vi "raster_scan_ground_shutter.vi"() -> ()   [LabVIEW 2013] (continued)
{"X"=1457.6770649491443, "Y"=0.9792905053235327}, {"X"=1458.7651269479165, "Y"=0.9823983446252466}, {"X"=1459.852974542116, "Y"=0.9830967304675241}, {"X"=1460.940607795108, "Y"=0.9785842230164021}, {"X"=1462.028026770236, "Y"=0.9775206880062371}, {"X"=1463.115231530815, "Y"=0.9787503056220913}, {"X"=1464.202222140141, "Y"=0.9797214290953251}, {"X"=1465.2889986614769, "Y"=0.9803641753236642}, {"X"=1466.3755611580664, "Y"=0.9821036191583837}, {"X"=1467.4619096931274, "Y"=0.978539694688825}, {"X"=1468.5480443298516, "Y"=0.9773624617620339}, {"X"=1469.6339651314086, "Y"=0.9807006551949096}, {"X"=1470.7196721609382, "Y"=0.9776792021711804}, {"X"=1471.8051654815604, "Y"=0.9801405710958422}, {"X"=1472.890445156365, "Y"=0.9788422567581777}, {"X"=1473.9755112484265, "Y"=0.9756071162075614}, {"X"=1475.0603638207806, "Y"=0.978305664540015}, {"X"=1476.1450029364496, "Y"=0.9757156870540381}, {"X"=1477.22942865843, "Y"=0.9787686258373013}, {"X"=1478.3136410496857, "Y"=0.9792534443330937}, {"X"=1479.3976401731636, "Y"=0.9761811767701299}, {"X"=1480.481426091784, "Y"=0.9801149830678351}, {"X"=1481.5649988684393, "Y"=0.9756151228933025}, {"X"=1482.6483585660003, "Y"=0.9791892417960691}, {"X"=1483.7315052473118, "Y"=0.9784822075875651}, {"X"=1484.8144389751922, "Y"=0.9803761026749522}, {"X"=1485.897159812443, "Y"=0.9794142210541505}, {"X"=1486.979667821831, "Y"=0.9777454282868382}, {"X"=1488.061963066103, "Y"=0.9765603212009248}, {"X"=1489.1440456079827, "Y"=0.9793187588636386}, {"X"=1490.2259155101667, "Y"=0.9805922827534587}, {"X"=1491.3075728353247, "Y"=0.9764488211952385}, {"X"=1492.3890176461057, "Y"=0.9783557981039106}, {"X"=1493.4702500051358, "Y"=0.9797315485802368}, {"X"=1494.5512699750122, "Y"=0.9776150196125559}, {"X"=1495.6320776183086, "Y"=0.9776877216361516}, {"X"=1496.712672997573, "Y"=0.9781695891128918}, {"X"=1497.7930561753328, "Y"=0.9738031398956338}, {"X"=1498.8732272140865, "Y"=0.975976844601347}, {"X"=1499.9531861763096, "Y"=0.9765304998861686}, {"X"=1501.0329331244568, "Y"=0.976932896128674}, {"X"=1502.1124681209478, "Y"=0.9800966831480284}, {"X"=1503.1917912281933, "Y"=0.9768824769343718}, {"X"=1504.2709025085678, "Y"=0.981309584860133}, {"X"=1505.3498020244213, "Y"=0.9788112290408383}, {"X"=1506.428489838087, "Y"=0.9749607521239584}, {"X"=1507.5069660118672, "Y"=0.9776436670703931}, {"X"=1508.5852306080433, "Y"=0.9781728498905934}, {"X"=1509.6632836888655, "Y"=0.9785040924428975}, {"X"=1510.7411253165735, "Y"=0.9808588594145039}, {"X"=1511.818755553368, "Y"=0.9802873517212242}, {"X"=1512.8961744614323, "Y"=0.9775486080858491}, {"X"=1513.973382102924, "Y"=0.9767280155604918}, {"X"=1515.0503785399785, "Y"=0.980209272149509}, {"X"=1516.1271638347032, "Y"=0.9800164628111341}, {"X"=1517.2037380491815, "Y"=0.9779781472644876}, {"X"=1518.2801012454781, "Y"=0.9801492617966195}, {"X"=1519.356253485624, "Y"=0.9786930631958413}, {"X"=1520.4321948316335, "Y"=0.9758135531220278}, {"X"=1521.507925345497, "Y"=0.9754907725499357}, {"X"=1522.5834450891723, "Y"=0.9781765485055535}, {"X"=1523.658754124602, "Y"=0.9787103618067179}, {"X"=1524.7338525137006, "Y"=0.9795724169903677}, {"X"=1525.8087403183565, "Y"=0.980684893431184}, {"X"=1526.8834176004366, "Y"=0.9771208914998462}, {"X"=1527.9578844217835, "Y"=0.9775073160780532}, {"X"=1529.032140844212, "Y"=0.9797555776149712}, {"X"=1530.10618692952, "Y"=0.975841176234859}, {"X"=1531.1800227394758, "Y"=0.9807727653780394}, {"X"=1532.2536483358228, "Y"=0.9802961901132733}, {"X"=1533.3270637802827, "Y"=0.9777395500524853}, {"X"=1534.400269134551, "Y"=0.9778205116075891}, {"X"=1535.4732644603034, "Y"=0.9790625062938085}, {"X"=1536.5460498191853, "Y"=0.9768981763432918}, {"X"=1537.6186252728232, "Y"=0.9786665184806389}, {"X"=1538.6909908828147, "Y"=0.9778748148771911}, {"X"=1539.7631467107403, "Y"=0.9774185537903284}, {"X"=1540.835092818148, "Y"=0.9794422669553383}, {"X"=1541.9068292665686, "Y"=0.9768522710498364}, {"X"=1542.9783561175022, "Y"=0.9779311791789327}, {"X"=1544.049673432434, "Y"=0.9777348271764831}, {"X"=1545.1207812728164, "Y"=0.9788311883596232}, {"X"=1546.1916797000786, "Y"=0.9801137926376271}, {"X"=1547.2623687756357, "Y"=0.9788638301844342}, {"X"=1548.3328485608647, "Y"=0.9773351540658165}, {"X"=1549.4031191171293, "Y"=0.9784129460538136}, {"X"=1550.473180505765, "Y"=0.9773105555519682}, {"X"=1551.543032788081, "Y"=0.9756165586699904}, {"X"=1552.6126760253678, "Y"=0.9806566212357941}, {"X"=1553.6821102788865, "Y"=0.9776974839417673}, {"X"=1554.7513356098798, "Y"=0.9798533480947225}, {"X"=1555.8203520795637, "Y"=0.9773735991839198}, {"X"=1556.8891597491306, "Y"=0.9781065565190785}, {"X"=1557.957758679745, "Y"=0.9791812863307896}, {"X"=1559.0261489325553, "Y"=0.976934001594789}, {"X"=1560.0943305686806, "Y"=0.9798934119983503}, {"X"=1561.1623036492178, "Y"=0.9797080714150074}, {"X"=1562.2300682352377, "Y"=0.9804595704839962}, {"X"=1563.2976243877897, "Y"=0.9780169362249083}, {"X"=1564.3649721679012, "Y"=0.9799845623788633}, {"X"=1565.432111636574, "Y"=0.9776505523367032}, {"X"=1566.4990428547812, "Y"=0.9786612468271689}, {"X"=1567.5657658834812, "Y"=0.9809144110707856}, {"X"=1568.6322807835995, "Y"=0.9757405630183322}, {"X"=1569.6985876160466, "Y"=0.9785541452864821}, {"X"=1570.7646864416984, "Y"=0.9818847727133657}, {"X"=1571.8305773214217, "Y"=0.9779227856602232}, {"X"=1572.896260316045, "Y"=0.9793508481684556}, {"X"=1573.9617354863833, "Y"=0.980887808587657}, {"X"=1575.027002893221, "Y"=0.9797121999265395}, {"X"=1576.0920625973235, "Y"=0.9795556996545292}, {"X"=1577.15691465943, "Y"=0.9766550361895545}, {"X"=1578.2215591402578, "Y"=0.9759789556077555}, {"X"=1579.2859961004988, "Y"=0.9815908904755111}, {"X"=1580.35022560082, "Y"=0.9785937882250549}, {"X"=1581.41424770187, "Y"=0.9819645665279645}, {"X"=1582.4780624642708, "Y"=0.979843167597932}, {"X"=1583.5416699486182, "Y"=0.9792802489088565}, {"X"=1584.6050702154869, "Y"=0.9790060313862785}, {"X"=1585.6682633254293, "Y"=0.9784271844295911}, {"X"=1586.7312493389722, "Y"=0.9784361245927183}, {"X"=1587.7940283166165, "Y"=0.9775708937146439}, {"X"=1588.856600318845, "Y"=0.9789041946582772}, {"X"=1589.9189654061154, "Y"=0.9774768633003437}, {"X"=1590.9811236388587, "Y"=0.9798817299531287}, {"X"=1592.0430750774847, "Y"=0.9768271507913547}, {"X"=1593.1048197823789, "Y"=0.9787911807962866}, {"X"=1594.1663578139055, "Y"=0.9783715358577475}, {"X"=1595.2276892324023, "Y"=0.9788361535376178}, {"X"=1596.2888140981859, "Y"=0.9793765834786251}, {"X"=1597.3497324715445, "Y"=0.9779362720028634}, {"X"=1598.410444412753, "Y"=0.9795457056765116}, {"X"=1599.4709499820517, "Y"=0.9797067699371061}, {"X"=1600.531249239662, "Y"=0.9808534483691963}, {"X"=1601.591342245785, "Y"=0.9781878073830106}, {"X"=1602.651229060596, "Y"=0.9802554323683685}, {"X"=1603.7109097442426, "Y"=0.9776897881450424}, {"X"=1604.7703843568543, "Y"=0.9797514273601062}, {"X"=1605.829652958537, "Y"=0.9789968213957626}, {"X"=1606.888715609371, "Y"=0.9786680583172949}, {"X"=1607.9475723694147, "Y"=0.9781996662549933}, {"X"=1609.006223298702, "Y"=0.9799905582549356}, {"X"=1610.0646684572441, "Y"=0.9801584266392093}, {"X"=1611.1229079050315, "Y"=0.9808165915061069}, {"X"=1612.1809417020254, "Y"=0.980629963941835}, {"X"=1613.2387699081667, "Y"=0.9779217757054299}, {"X"=1614.2963925833749, "Y"=0.980291231246423}, {"X"=1615.353809787546, "Y"=0.9802126966035473}, {"X"=1616.4110215805492, "Y"=0.9806800387009521}, {"X"=1617.468028022235, "Y"=0.9825340406943407}, {"X"=1618.5248291724251, "Y"=0.9788256639790675}, {"X"=1619.5814250909243, "Y"=0.9802906842015114}, {"X"=1620.637815837509, "Y"=0.979685976141551}, {"X"=1621.6940014719337, "Y"=0.9800339027601165}, {"X"=1622.7499820539335, "Y"=0.9779521660841378}, {"X"=1623.8057576432159, "Y"=0.9793762038551321}, {"X"=1624.8613282994656, "Y"=0.9785756484834109}, {"X"=1625.9166940823447, "Y"=0.9772795374000064}, {"X"=1626.971855051495, "Y"=0.9780014724416649}, {"X"=1628.0268112665321, "Y"=0.9769491921287421}, {"X"=1629.0815627870463, "Y"=0.981333694440951}, {"X"=1630.136109672612, "Y"=0.9784390781431715}, {"X"=1631.1904519827697, "Y"=0.9790742732109099}, {"X"=1632.2445897770504, "Y"=0.9796612246815406}, {"X"=1633.2985231149485, "Y"=0.9779598916744058}, {"X"=1634.3522520559459, "Y"=0.9772464628134946}, {"X"=1635.4057766594958, "Y"=0.9793400653452339}, {"X"=1636.4590969850296, "Y"=0.9797116577597221}, {"X"=1637.5122130919533, "Y"=0.9797059940747953}, {"X"=1638.5651250396568, "Y"=0.9808562777149027}, {"X"=1639.6178328874985, "Y"=0.9790804555327355}, {"X"=1640.6703366948186, "Y"=0.9788362371686626}, {"X"=1641.722636520934, "Y"=0.9787844420078925}, {"X"=1642.7747324251397, "Y"=0.9794474398454981}, {"X"=1643.8266244667045, "Y"=0.9804131255057831}, {"X"=1644.878312704874, "Y"=0.9768249479329455}, {"X"=1645.9297971988753, "Y"=0.9799389865441378}, {"X"=1646.9810780079088, "Y"=0.9783432068536082}, {"X"=1648.0321551911518, "Y"=0.9775263305205893}, {"X"=1649.083028807763, "Y"=0.9787347803249032}, {"X"=1650.1336989168726, "Y"=0.9808567682226018}, {"X"=1651.184165577591, "Y"=0.9782522449877368}, {"X"=1652.2344288490056, "Y"=0.9789066233804873}, {"X"=1653.284488790181, "Y"=0.978399712160505}, {"X"=1654.334345460157, "Y"=0.9775518534383865}, {"X"=1655.3839989179503, "Y"=0.9776201692032794}, {"X"=1656.4334492225616, "Y"=0.9790505282699306}, {"X"=1657.4826964329582, "Y"=0.9791007362859836}, {"X"=1658.5317406080926, "Y"=0.9796289092089305}, {"X"=1659.5805818068911, "Y"=0.9802344480197129}, {"X"=1660.6292200882588, "Y"=0.9794118671835017}, {"X"=1661.6776555110757, "Y"=0.9769578407595142}, {"X"=1662.725888134202, "Y"=0.9796671523854356}, {"X"=1663.7739180164745, "Y"=0.9772899941448419}, {"X"=1664.8217452167003, "Y"=0.9789999657090263}, {"X"=1665.869369793676, "Y"=0.9793822552018605}, {"X"=1666.9167918061676, "Y"=0.9778192616893263}, {"X"=1667.9640113129212, "Y"=0.9777885231437959}, {"X"=1669.0110283726551, "Y"=0.9797417352632923}, {"X"=1670.0578430440723, "Y"=0.9809342630258361}, {"X"=1671.104455385848, "Y"=0.9779252084439294}, {"X"=1672.1508654566371, "Y"=0.9766078448496384}, {"X"=1673.1970733150715, "Y"=0.9799766985367611}, {"X"=1674.2430790197561, "Y"=0.9784335113759398}, {"X"=1675.2888826292817, "Y"=0.9792316725161806}, {"X"=1676.3344842022125, "Y"=0.976438469155643}, {"X"=1677.3798837970842, "Y"=0.9789431735090179}, {"X"=1678.4250814724203, "Y"=0.9784990647101345}, {"X"=1679.4700772867131, "Y"=0.9784634992400977}, {"X"=1680.5148712984362, "Y"=0.9757776031845267}, {"X"=1681.5594635660389, "Y"=0.9785753222902629}, {"X"=1682.603854147955, "Y"=0.9762430899631663}, {"X"=1683.648043102582, "Y"=0.9786154222348789}, {"X"=1684.6920304883088, "Y"=0.982601098721033}, {"X"=1685.735816363493, "Y"=0.9787598651333007}, {"X"=1686.779400786472, "Y"=0.9796236090165618}, {"X"=1687.8227838155622, "Y"=0.9807569854592928}, {"X"=1688.865965509057, "Y"=0.9777286147683862}, {"X"=1689.9089459252239, "Y"=0.979530268059855}, {"X"=1690.9517251223103, "Y"=0.9795518390335218}, {"X"=1691.9943031585465, "Y"=0.9762685981835564}, {"X"=1693.0366800921304, "Y"=0.9764990724345295}, {"X"=1694.0788559812445, "Y"=0.9793632033260535}, {"X"=1695.1208308840478, "Y"=0.9784431206603648}, {"X"=1696.162604858673, "Y"=0.9800970609348729}, {"X"=1697.204177963233, "Y"=0.9798274514050527}, {"X"=1698.2455502558198, "Y"=0.9767392079564985}, {"X"=1699.2867217945052, "Y"=0.9779580128194008}, {"X"=1700.3276926373287, "Y"=0.9756815094964185}, {"X"=1701.368462842319, "Y"=0.9800487876203458}, {"X"=1702.4090324674746, "Y"=0.9761434590853568}, {"X"=1703.4494015707742, "Y"=0.9778648023676554}, {"X"=1704.4895702101746, "Y"=0.9774400128118678}, {"X"=1705.5295384436095, "Y"=0.9787943730431603}, {"X"=1706.5693063289923, "Y"=0.978395003858087}, {"X"=1707.6088739242089, "Y"=0.9781690442984677}, {"X"=1708.6482412871314, "Y"=0.9768357067469553}, {"X"=1709.6874084756023, "Y"=0.9785722403014319}, {"X"=1710.7263755474444, "Y"=0.9794128983222802}, {"X"=1711.765142560456, "Y"=0.9762472144277007}, {"X"=1712.8037095724192, "Y"=0.980017853288302}, {"X"=1713.8420766410868, "Y"=0.9784777089298898}, {"X"=1714.8802438241908, "Y"=0.9788070467014609}, {"X"=1715.918211179447, "Y"=0.9777741715615405}, {"X"=1716.9559787645442, "Y"=0.9791586404821226}, {"X"=1717.9935466371467, "Y"=0.9797751943038832}, {"X"=1719.0309148548993, "Y"=0.9781731952451092}, {"X"=1720.068083475427, "Y"=0.9786903221799141}, {"X"=1721.1050525563276, "Y"=0.9772549072141031}, {"X"=1722.1418221551803, "Y"=0.9765150697236492}, {"X"=1723.1783923295413, "Y"=0.9773240982124607}, {"X"=1724.214763136945, "Y"=0.9791583881092693}, {"X"=1725.250934634904, "Y"=0.9784526724453544}, {"X"=1726.2869068809046, "Y"=0.9777962347228817}, {"X"=1727.3226799324184, "Y"=0.9780085659065672}, {"X"=1728.3582538468886, "Y"=0.9779903185671098}, {"X"=1729.393628681741, "Y"=0.9766604181863742}, {"X"=1730.428804494373, "Y"=0.9791432873661055}, {"X"=1731.4637813421655, "Y"=0.9798748523350176}, {"X"=1732.4985592824764, "Y"=0.9784743079655346}, {"X"=1733.5331383726434, "Y"=0.9784825300354543}, {"X"=1734.5675186699748, "Y"=0.9785467117994335}, {"X"=1735.6017002317642, "Y"=0.979534546347603}, {"X"=1736.6356831152796, "Y"=0.982177067294777}, {"X"=1737.6694673777704, "Y"=0.9797240911901233}, {"X"=1738.7030530764594, "Y"=0.9790253743667566}, {"X"=1739.7364402685507, "Y"=0.9815129154446102}, {"X"=1740.7696290112233, "Y"=0.980432858830974}, {"X"=1741.8026193616408, "Y"=0.9798457306402057}, {"X"=1742.835411376938, "Y"=0.9781409027568759}, {"X"=1743.868005114229, "Y"=0.9788862198138762}, {"X"=1744.9004006306095, "Y"=0.9757087423855413}, {"X"=1745.9325979831483, "Y"=0.9798092930085314}, {"X"=1746.9645972288977, "Y"=0.9789802741859566}, {"X"=1747.9963984248845, "Y"=0.9805471172994134}, {"X"=1749.0280016281145, "Y"=0.9785389300564209}, {"X"=1750.0594068955684, "Y"=0.9770374391897149}, {"X"=1751.0906142842127, "Y"=0.9775021384461788}, {"X"=1752.1216238509876, "Y"=0.9794676904895196}, {"X"=1753.152435652809, "Y"=0.9801654916078579}, {"X"=1754.183049746574, "Y"=0.9789424499526841}, {"X"=1755.2134661891573, "Y"=0.9770892255789045}, {"X"=1756.243685037413, "Y"=0.9776593168216676}, {"X"=1757.2737063481677, "Y"=0.9779906119034862}, {"X"=1758.3035301782381, "Y"=0.9781764711339365}, {"X"=1759.3331565844067, "Y"=0.9796097506756954}, {"X"=1760.3625856234391, "Y"=0.9788229781819409}, {"X"=1761.3918173520813, "Y"=0.9797000451931207}, {"X"=1762.4208518270536, "Y"=0.9772262704494723}, {"X"=1763.449689105058, "Y"=0.9793011383686007}, {"X"=1764.4783292427744, "Y"=0.9797462455262113}, {"X"=1765.5067722968568, "Y"=0.9790906455724389}, {"X"=1766.5350183239393, "Y"=0.9787694192292369}, {"X"=1767.5630673806413, "Y"=0.9773923919944699}, {"X"=1768.5909195235492, "Y"=0.9780613554354805}, {"X"=1769.6185748092373, "Y"=0.9753480333886292}, {"X"=1770.6460332942527, "Y"=0.9776669800733908}, {"X"=1771.6732950351213, "Y"=0.9774852126882629}, {"X"=1772.7003600883502, "Y"=0.9792762661382732}, {"X"=1773.727228510419, "Y"=0.9778884418100252}, {"X"=1774.7539003577956, "Y"=0.9758349135196726}, {"X"=1775.780375686917, "Y"=0.9790951870913759}, {"X"=1776.8066545542008, "Y"=0.9784810089527837}, {"X"=1777.832737016047, "Y"=0.9797035920414627}, {"X"=1778.8586231288302, "Y"=0.9794844663168093}, {"X"=1779.8843129489044, "Y"=0.9781376071318827}, {"X"=1780.9098065326032, "Y"=0.9750094677165442}, {"X"=1781.9351039362352, "Y"=0.9780984964063493}, {"X"=1782.9602052160903, "Y"=0.9754901241953642}, {"X"=1783.9851104284364, "Y"=0.9788789968076032}, {"X"=1785.0098196295219, "Y"=0.9761625032883274}, {"X"=1786.0343328755714, "Y"=0.977184310500348}, {"X"=1787.0586502227857, "Y"=0.9763453938178065}, {"X"=1788.0827717273478, "Y"=0.9792373851417304}, {"X"=1789.1066974454172, "Y"=0.9754176689748405}, {"X"=1790.1304274331344, "Y"=0.9787418979212442}, {"X"=1791.1539617466153, "Y"=0.9779537906626933}, {"X"=1792.1773004419586, "Y"=0.9783783911467727}, {"X"=1793.200443575237, "Y"=0.9777594296522633}, {"X"=1794.2233912025015, "Y"=0.9773798356027293}, {"X"=1795.2461433797885, "Y"=0.9772880946873316}, {"X"=1796.268700163103, "Y"=0.976721049350884}, {"X"=1797.291061608438, "Y"=0.9782575538452549}, {"X"=1798.3132277717596, "Y"=0.981480761676852}, {"X"=1799.3351987090107, "Y"=0.9767565408104497}, {"X"=1800.356974476123, "Y"=0.9764783426267764}, {"X"=1801.3785551289936, "Y"=0.9783902648770324}, {"X"=1802.3999407235092, "Y"=0.9785140953183166}, {"X"=1803.4211313155251, "Y"=0.9775113160777504}, {"X"=1804.4421269608847, "Y"=0.9785064598563911}, {"X"=1805.462927715407, "Y"=0.9778236195481496}, {"X"=1806.4835336348847, "Y"=0.9778192965434114}, {"X"=1807.503944775096, "Y"=0.978177936326559}, {"X"=1808.5241611917927, "Y"=0.9786243269548447}, {"X"=1809.5441829407114, "Y"=0.9795102802219587}, {"X"=1810.5640100775604, "Y"=0.977832296174399}, {"X"=1811.5836426580333, "Y"=0.9801041553279659}, {"X"=1812.6030807377952, "Y"=0.9787686082046061}, {"X"=1813.622324372498, "Y"=0.9762591413703259}, {"X"=1814.6413736177635, "Y"=0.9785764588841125}, {"X"=1815.6602285292006, "Y"=0.9778338211092795}, {"X"=1816.678889162394, "Y"=0.9786470411846112}, {"X"=1817.6973555729046, "Y"=0.9780455869984812}, {"X"=1818.7156278162763, "Y"=0.9772685688395546}, {"X"=1819.7337059480287, "Y"=0.9790073728881996}, {"X"=1820.7515900236604, "Y"=0.9776787156291022}, {"X"=1821.7692800986495, "Y"=0.981571042496983}, {"X"=1822.7867762284554, "Y"=0.9781551040759343}, {"X"=1823.8040784685134, "Y"=0.9775827328985149}, {"X"=1824.821186874237, "Y"=0.9790314094428728}, {"X"=1825.8381015010223, "Y"=0.97651494318833}, {"X"=1826.8548224042418, "Y"=0.98117111940764}, {"X"=1827.8713496392438, "Y"=0.9790448337557365}, {"X"=1828.8876832613619, "Y"=0.9792762568727814}, {"X"=1829.9038233259057, "Y"=0.9814170280977215}, {"X"=1830.9197698881605, "Y"=0.9769394138414527}, {"X"=1831.9355230033968, "Y"=0.9779927873623165}, {"X"=1832.9510827268593, "Y"=0.9795814602795806}, {"X"=1833.966449113775, "Y"=0.9813169438214728}, {"X"=1834.9816222193472, "Y"=0.9791962839304864}, {"X"=1835.9966020987592, "Y"=0.978443602610066}, {"X"=1837.0113888071735, "Y"=0.979330901923164}, {"X"=1838.025982399728, "Y"=0.9793733883949935}, {"X"=1839.040382931546, "Y"=0.9785176881927857}, {"X"=1840.0545904577286, "Y"=0.9787976042022226}, {"X"=1841.068605033351, "Y"=0.9794191523481688}, {"X"=1842.0824267134715, "Y"=0.9790665855910927}, {"X"=1843.0960555531262, "Y"=0.9783607833794199}, {"X"=1844.1094916073316, "Y"=0.981239000018723}, {"X"=1845.1227349310811, "Y"=0.9760725103032508}, {"X"=1846.1357855793499, "Y"=0.9802543813509697}, {"X"=1847.1486436070877, "Y"=0.9802118944100315}, {"X"=1848.1613090692265, "Y"=0.9788447902308257}, {"X"=1849.1737820206813, "Y"=0.9788741535108112}, {"X"=1850.1860625163386, "Y"=0.9797346774488815}, {"X"=1851.19815061107, "Y"=0.9769856196301054}, {"X"=1852.2100463597233, "Y"=0.979878008180614}, {"X"=1853.221749817122, "Y"=0.9761372153962043}, {"X"=1854.233261038079, "Y"=0.9790780443105339}, {"X"=1855.2445800773748, "Y"=0.9786918992409724}, {"X"=1856.2557069897791, "Y"=0.9783276499689203}, {"X"=1857.2666418300307, "Y"=0.9797503315777013}, {"X"=1858.2773846528562, "Y"=0.9776083716249421}, {"X"=1859.2879355129598, "Y"=0.9770551335500846}, {"X"=1860.2982944650225, "Y"=0.979004766786602}, {"X"=1861.3084615637028, "Y"=0.9799782313870046}, {"X"=1862.3184368636428, "Y"=0.9770803550491507}, {"X"=1863.3282204194622, "Y"=0.978975563881147}, {"X"=1864.337812285757, "Y"=0.9799645707401039}, {"X"=1865.3472125171106, "Y"=0.9801723270677862}, {"X"=1866.3564211680773, "Y"=0.9788358662998463}, {"X"=1867.3654382931952, "Y"=0.9765847371482588}, {"X"=1868.3742639469779, "Y"=0.9790676397118934}, {"X"=1869.3828981839238, "Y"=0.9812889246294414}, {"X"=1870.391341058503, "Y"=0.9774577161709844}, {"X"=1871.3995926251753, "Y"=0.980594262876655}, {"X"=1872.4076529383697, "Y"=0.9792702411654549}, {"X"=1873.4155220524979, "Y"=0.9790746036664525}, {"X"=1874.4232000219565, "Y"=0.9810852257689248}, {"X"=1875.4306869011118, "Y"=0.9795606590451479}, {"X"=1876.4379827443195, "Y"=0.9801611141715787}, {"X"=1877.4450876059084, "Y"=0.9786582015465105}, {"X"=1878.4520015401865, "Y"=0.9788312536969757}, {"X"=1879.4587246014419, "Y"=0.9795506376816854}, {"X"=1880.4652568439433, "Y"=0.9808280442755959}, {"X"=1881.4715983219419, "Y"=0.9782914192105046}, {"X"=1882.4777490896631, "Y"=0.9795263525003457}, {"X"=1883.4837092013126, "Y"=0.9802605203766053}, {"X"=1884.4894787110768, "Y"=0.9801816775097535}, {"X"=1885.4950576731223, "Y"=0.9801096012430007}, {"X"=1886.5004461415922, "Y"=0.9796802539288852}, {"X"=1887.5056441706138, "Y"=0.9788520860491313}, {"X"=1888.510651814289, "Y"=0.978659668379837}, {"X"=1889.5154691267023, "Y"=0.977015575532349}, {"X"=1890.5200961619184, "Y"=0.9787515604122116}, {"X"=1891.524532973976, "Y"=0.9768297562113655}, {"X"=1892.5287796169011, "Y"=0.9785475232918758}, {"X"=1893.5328361446932, "Y"=0.978116773405777}, {"X"=1894.5367026113352, "Y"=0.9811734737768301}, {"X"=1895.540379070785, "Y"=0.9804007166695333}, {"X"=1896.5438655769865, "Y"=0.9802706286345342}, {"X"=1897.547162183857, "Y"=0.9789474999633454}, {"X"=1898.5502689452985, "Y"=0.9764637671130718}, {"X"=1899.5531859151895, "Y"=0.9778795664386171}, {"X"=1900.5559131473867, "Y"=0.9784828326256647}, {"X"=1901.5584506957314, "Y"=0.9787769985370004}, {"X"=1902.5607986140392, "Y"=0.9798369721889083}, {"X"=1903.5629569561104, "Y"=0.9820482127941871}, {"X"=1904.5649257757213, "Y"=0.9785111601732347}, {"X"=1905.5667051266269, "Y"=0.9796830451602337}, {"X"=1906.5682950625664, "Y"=0.9787209677077426}, {"X"=1907.5696956372535, "Y"=0.98122288862003}, {"X"=1908.570906904389, "Y"=0.9809305064389832}, {"X"=1909.5719289176448, "Y"=0.9790387967034756}, {"X"=1910.5727617306782, "Y"=0.9794775159709218}, {"X"=1911.5734053971228, "Y"=0.9807386672057676}, {"X"=1912.573859970592, "Y"=0.9779631608593421}, {"X"=1913.574125504687, "Y"=0.9802046696643638}, {"X"=1914.5742020529756, "Y"=0.9780746838834492}, {"X"=1915.5740896690154, "Y"=0.9808649271816879}, {"X"=1916.573788406338, "Y"=0.9804333729213841}, {"X"=1917.5732983184594, "Y"=0.9801111109332562}, {"X"=1918.5726194588722, "Y"=0.9782040652735418}, {"X"=1919.5717518810488, "Y"=0.9791773277008486}, {"X"=1920.5706956384452, "Y"=0.9796555558287696}, {"X"=1921.5694507844885, "Y"=0.9789302800714461}, {"X"=1922.5680173725973, "Y"=0.9815528643924064}, {"X"=1923.566395456162, "Y"=0.9778044788192052}, {"X"=1924.5645850885558, "Y"=0.9783244097180387}, {"X"=1925.5625863231303, "Y"=0.9778964226146003}, {"X"=1926.5603992132171, "Y"=0.9787447398864959}, {"X"=1927.5580238121288, "Y"=0.9811759269001352}, {"X"=1928.5554601731558, "Y"=0.9798108032783646}, {"X"=1929.552708349572, "Y"=0.9798681796090567}, {"X"=1930.5497683946285, "Y"=0.9788799727761672}, {"X"=1931.5466403615578, "Y"=0.9788770140009356}, {"X"=1932.543324303568, "Y"=0.9799177632065718}, {"X"=1933.5398202738547, "Y"=0.9799634201036204}, {"X"=1934.5361283255868, "Y"=0.9798222448100651}, {"X"=1935.5322485119166, "Y"=0.9808393976744711}, {"X"=1936.528180885976, "Y"=0.9816005991663963}, {"X"=1937.523925500872, "Y"=0.97864600755322}, {"X"=1938.519482409702, "Y"=0.980309985973617}, {"X"=1939.5148516655336, "Y"=0.9781692490184501}, {"X"=1940.5100333214207, "Y"=0.9785093256720591}, {"X"=1941.5050274303896, "Y"=0.9799035052070364}, {"X"=1942.4998340454558, "Y"=0.9780111452063708}, {"X"=1943.4944532196087, "Y"=0.9817768573475947}, {"X"=1944.4888850058198, "Y"=0.9782104729191251}, {"X"=1945.483129457042, "Y"=0.979143828287662}, {"X"=1946.4771866262035, "Y"=0.9782644829264983}, {"X"=1947.471056566218, "Y"=0.97950360852036}, {"X"=1948.4647393299792, "Y"=0.9783169772597466}, {"X"=1949.4582349703528, "Y"=0.9798836359151304}, {"X"=1950.451543540196, "Y"=0.9791266953634022}, {"X"=1951.4446650923376, "Y"=0.9789837971330411}, {"X"=1952.4375996795911, "Y"=0.9813588982417887}, {"X"=1953.4303473547443, "Y"=0.9790520184393244}, {"X"=1954.422908170576, "Y"=0.9815722723554481}, {"X"=1955.415282179835, "Y"=0.9784927175757242}, {"X"=1956.4074694352523, "Y"=0.9788729195898936}, {"X"=1957.399469989544, "Y"=0.9791868614295317}, {"X"=1958.3912838953984, "Y"=0.9808439674180319}, {"X"=1959.382911205492, "Y"=0.9794424127876905}, {"X"=1960.3743519724785, "Y"=0.9811556122378184}, {"X"=1961.3656062489868, "Y"=0.9808021942940341}, {"X"=1962.3566740876313, "Y"=0.9800973819614038}, {"X"=1963.347555541011, "Y"=0.9795272574137769}, {"X"=1964.3382506616945, "Y"=0.9788140858856408}, {"X"=1965.3287595022373, "Y"=0.9780253232029532}, {"X"=1966.3190821151757, "Y"=0.979245748551627}, {"X"=1967.3092185530195, "Y"=0.9777558477121077}, {"X"=1968.2991688682703, "Y"=0.980276730191531}, {"X"=1969.288933113397, "Y"=0.9799821956293429}, {"X"=1970.2785113408574, "Y"=0.978955057838978}, {"X"=1971.2679036030884, "Y"=0.9823503552134017}, {"X"=1972.2571099525062, "Y"=0.9793230769314857}, {"X"=1973.246130441504, "Y"=0.9805669908359534}, {"X"=1974.234965122462, "Y"=0.9781158302205418}, {"X"=1975.223614047734, "Y"=0.9775909120825961}, {"X"=1976.212077269661, "Y"=0.979277706163912}, {"X"=1977.2003548405555, "Y"=0.9800070006509044}, {"X"=1978.1884468127198, "Y"=0.9795861716333901}, {"X"=1979.1763532384293, "Y"=0.977022092442501}, {"X"=1980.1640741699453, "Y"=0.9789258844658819}, {"X"=1981.1516096595064, "Y"=0.9792859180687412}, {"X"=1982.1389597593302, "Y"=0.9796248230956071}, {"X"=1983.1261245216187, "Y"=0.9804563919160044}, {"X"=1984.1131039985503, "Y"=0.979893234963858}, {"X"=1985.0998982422836, "Y"=0.9788294025328086}, {"X"=1986.086507304967, "Y"=0.9769723734116809}, {"X"=1987.0729312387155, "Y"=0.9783824752784152}, {"X"=1988.0591700956336, "Y"=0.9792177578466847}, {"X"=1989.0452239278025, "Y"=0.9788646746877344}, {"X"=1990.0310927872854, "Y"=0.9797103022782087}, {"X"=1991.0167767261282, "Y"=0.9786557517258911}, {"X"=1992.0022757963511, "Y"=0.9784247299328789}, {"X"=1992.987590049959, "Y"=0.9799351881103269}, {"X"=1993.9727195389369, "Y"=0.9801767642340488}, {"X"=1994.957664315253, "Y"=0.9791864057834342}, {"X"=1995.942424430849, "Y"=0.9806157724480351}, {"X"=1996.9269999376543, "Y"=0.9814342305423074}, {"X"=1997.9113908875738, "Y"=0.979347148988982}, {"X"=1998.8955973324953, "Y"=0.9787358726657928}, {"X"=1999.8796193242888, "Y"=0.9799108384264307}, {"X"=2000.8634569147994, "Y"=0.9801913761237805}, {"X"=2001.8471101558578, "Y"=0.9806815968287386}, {"X"=2002.8305790992738, "Y"=0.9791286421943739}]
  in  "# Images":u16=200 min=2 max=10000 step=2
  out "error out":errorcluster
  out "Camera Handle":u32=16842752
  out "Temperature":dbl=-75.5
  in  "error in":errorcluster
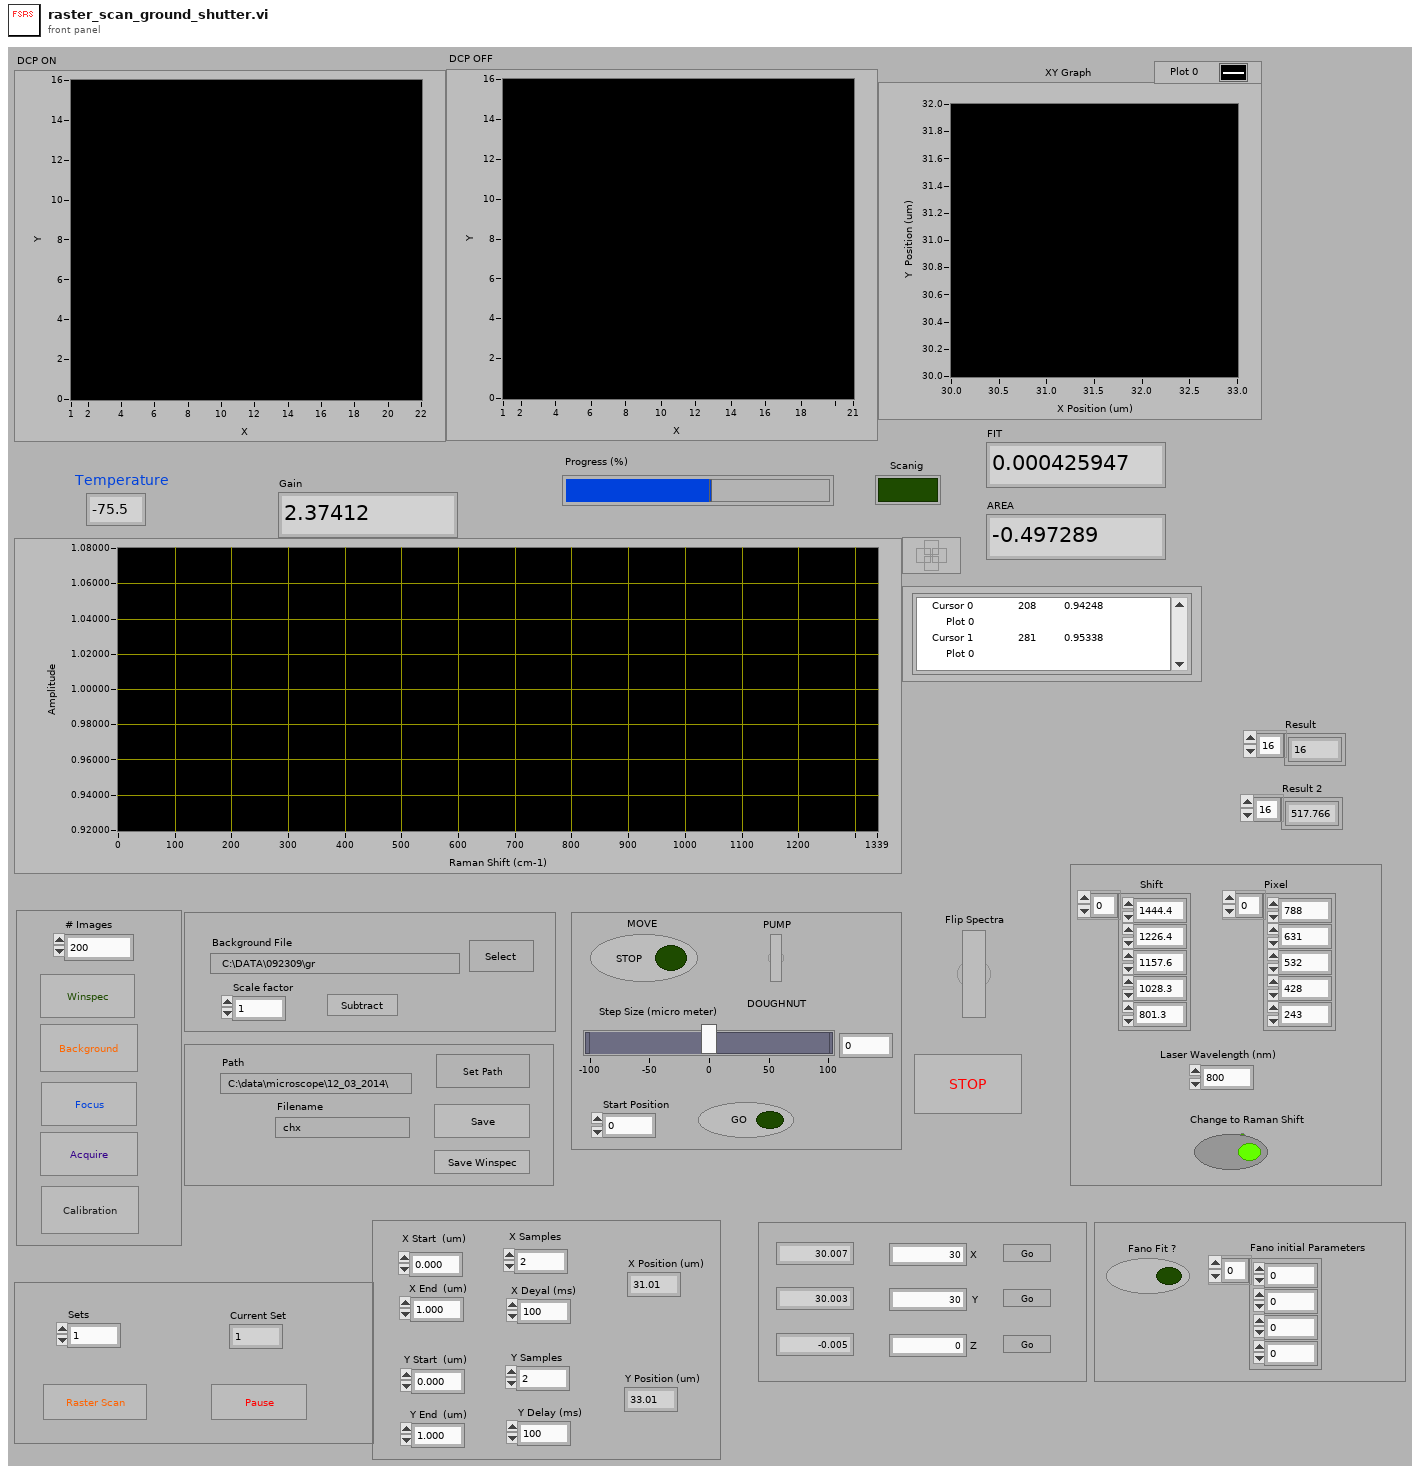
[diagram p1: front panel]
types:
  T1 = typedef "Control 2.ctl" = dbl[]
  T2 = cluster{"X start":u32, "X end":u32, "X Binning/Grouping":u32, "Y start":u32, "Y end":u32, "Y Binning/Grouping":u32}
  T3 = cluster{dbl[][], dbl[][], dbl[][], dbl[][], bool}
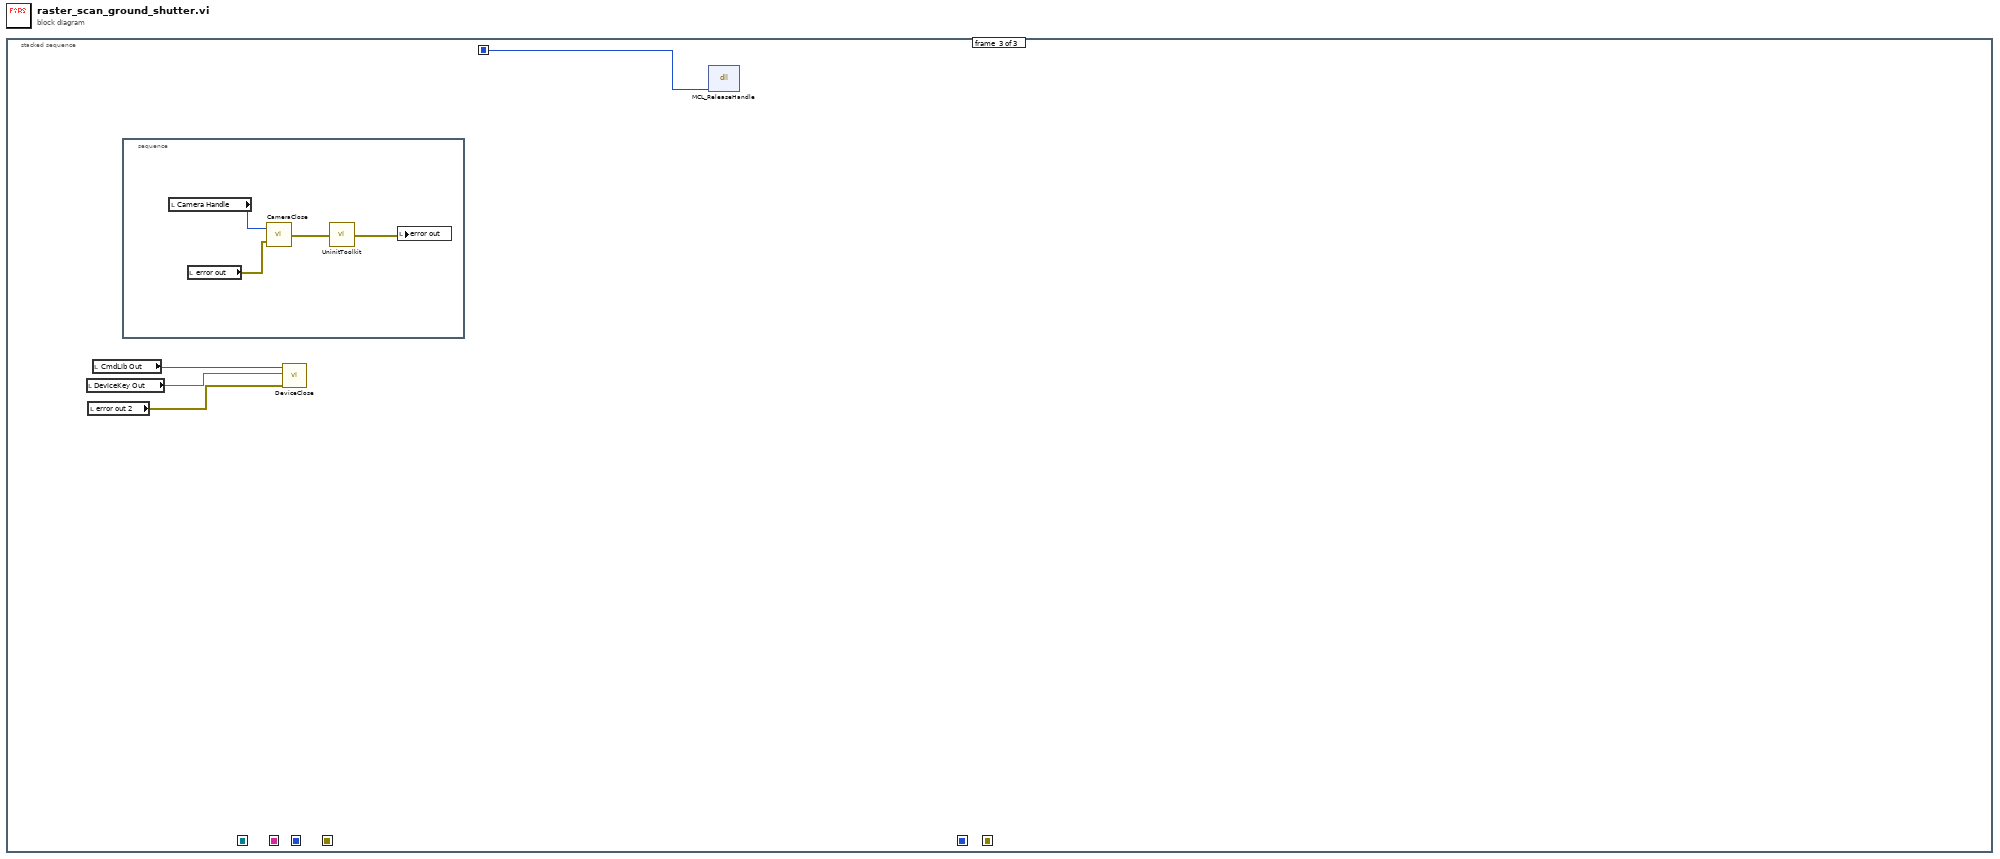
[diagram p0: block diagram]
diagram:
  n1 = stacked-sequence {
    seq-local: [w9 _ _] -> [_ w101 _]
    seq-local: [w8 _ _] -> [_ w100 _]
    seq-local: [w7 _ _] -> [_ w99 _]
    seq-local: [w6 _ _] -> [_ w98 _]
    seq-local: [w5 _ _] -> [_ w97 w744]
    seq-local: [w4 _ _] -> [_ w96 _]
    seq-local: [w3 _ _] -> [_ w95 _]
    frame #0 {
      w1 = 1340
      w67 = 0
      w69 = 8
      # "4: shutter opened while waiting for trigger\n3: Shutter opened during entire acq sequence\n2:Shutter opened and closed for each exposure\n\nOther numbers: Time in ms to open and close"
      # "1 is for free run, 3 ext sync"
      # "Parameter id settings:\n119: enable custon timing for horizontal and vertical shift\n121:Parallel shift time override\n146: Skip serial register clean\n 4:  Set logic output to \"Not Ready\" (necessary for chopper sync)"
      # "Setting up the PIXIS and all the environment variables\nHave Renee fill in the rest."
      n2 = call "ExSubInitNOpenCam.vi"("error in (no error)"="error in") -> ("Camera Handle"=w82:u32, "error out"=w39:errorcluster)
      n3 = call <userlib>:"CameraGetDataDim.vi"("Camera Handle"=w82, "error in"=w39) -> ("Camera Handle"=w79:u32, "Xdim"=w81:u32, "Ydim"=w80:u32, "error out"=w78:errorcluster)
      n4 = global write "MaxX.vi" "X Max in"(w81) -> ()
      n5 = global write "MaxY.vi" "Max Y in"(w80) -> ()
      n6 = call "pico_init.vi"() -> ("error out 3"=w6:errorcluster, "ID"=w7:i32, "key"=w8:string, "CmdLib Out"=w9:refnum<k24>)  [unwired: 8 in]
      n7 = call <userlib>:"CameraSetTemp.vi"("error in (no error)"=w78, "Temperature"=-75, "Camera Handle"=w79) -> ("error out"=w75:errorcluster, "Camera Handle"=w76:u32)
      n8 = call <userlib>:"CameraADCset.vi"("ADC offset"=0, "Read Out port"=2, "error in (no error)"=w75, "ADC Gain"=1, "ADC Speed"=-2, "Camera Handle"=w76) -> ("error out"=w70:errorcluster, "Camera Handle"=w71:u32)
      n9 = Bundle(w69, w69, 100, w67, w67, w1) -> (w66:cluster{i32, i32, i32, i32, i32, i32})  [unwired: 1 in]
      n10 = call <userlib>:"CameraSetCustomChip.vi"("error in (no error)"=w70, "Custom Chip Settings"=w66, "Enable/Disable Custom Chip"=TRUE, "Camera Handle"=w71) -> ("error out"=w63:errorcluster, "Camera Handle"=w64:u32)
      n11 = call <userlib>:"CameraSkips.vi"("Camera Handle"=w64, "Minimum Block Size"=100, "Number of Minimum blocks"=1, "error in"=w63, "Type of Skips"=1) -> ("Camera Handle"=w58:u32, "error out"=w59:errorcluster)
      n12 = call "StandardInit.vi"() -> ("Outgoing Handle"=w5:i32)  [unwired: 1 in]
      n13 = call <userlib>:"CameraCleans.vi"("Camera Handle"=w58, "Number of Clears"=1, "Number of Strips Per Clear"=100, "error in"=w59, "Continuous Clears"=0) -> ("Camera Handle"=w53:u32, "error out"=w54:errorcluster)
      n14 = call <userlib>:"CameraTrigger.vi"("error in"=w54, "Trigger Edge"=1, "Timing Mode"=3, "Camera Handle"=w53) -> ("error out"=w31:errorcluster, "Camera Handle"=w30:u32)
      n15 = Bundle By Name(cluster=T2 {"X start"=0, "X end"=0, "X Binning/Grouping"=0, "Y start"=0, "Y end"=0, "Y Binning/Grouping"=0} ("ROI Params"), "X start"=u32 1, "X end"=u32 1340, "X Binning/Grouping"=u32 1, "Y start"=u32 1, "Y end"=u32 100, "Y Binning/Grouping"=u32 100) -> (w12:T2)
      n16 = call <userlib>:"CameraROI.vi"("error in"=w31, "ROI Params"=w12, "ROI Index"=1, "Camera Handle"=w30) -> ("error out"=w25:errorcluster, "Camera Handle"=w24:u32)
      n17 = call <userlib>:"CameraShutter.vi"("Camera Handle"=w24, "Shutter Comp Time: Pre Open"=0, "Shutter Comp Time: Post Open"=0, "error in"=w25, "Shutter State"=3) -> ("Camera Handle"=w23:u32, "error out"=w14:errorcluster)
      n18 = call <userlib>:"CameraSetVar.vi"("error in"=w14, "Value"=1.0, "Parameter ID"=119, "Camera Handle"=w23) -> ("error out"=w48:errorcluster, "CameraHandle"=w46:u32)
      n19 = call <userlib>:"CameraSetVar.vi"("error in"=w48, "Value"=3200.0, "Parameter ID"=121, "Camera Handle"=w46) -> ("error out"=w47:errorcluster, "CameraHandle"=w45:u32)
      n20 = call <userlib>:"CameraSetVar.vi"("error in"=w47, "Value"=1.0, "Parameter ID"=146, "Camera Handle"=w45) -> ("error out"=w19:errorcluster, "CameraHandle"=w18:u32)
      n21 = call <userlib>:"CameraSetVar.vi"("error in"=w19, "Value"=3.0, "Parameter ID"=4, "Camera Handle"=w18) -> ("error out"=w17:errorcluster, "CameraHandle"=w10:u32)
      n22 = call <userlib>:"ToolKitIsError.vi"("error in"=w17, "Reserved"=w10) -> ("error out"=w49:errorcluster, "Error Flag"=w50:bool)
      n23 = case shown="False" w50 {
        tunnel: w49 -> [_ w94]
        tunnel: [w93 w94] -> w11
        tunnel: w39 -> [w93 _]
        frame False {
        }
        frame True {
        }
      }
      n24 = while {
        tunnel: w11 -> [w91]
        tunnel: [w90] -> w27
        tunnel: w10 -> [w89]
        tunnel: [w88] -> w28
        stop <- w86 continue-if-true
        # "This loop makes sure the camera has cooled down completely"
        n25 = call <userlib>:"CameraGetTemp.vi"("Camera Handle"=w89, "error in (no error)"=w91) -> ("Camera Handle"=w88:u32, "Temperature"=w85:dbl, "error out"=w90:errorcluster)
        "Temperature" <- w85
        n26 = Wait Until Next ms Multiple(millisecond multiple=1000 ("ADC Gain")) -> ()  [unwired: 1 out]
        n27 = Greater?(x=w85, y=-75) -> (0:w86:bool)
      }
      "Camera Handle" <- w28
      "error out" <- w27
      n28 = for {
        N: w1 -> [_]
        tunnel: [w84] -> w2 mode=indexing
        i -> [w84]
      }
      n29 = local write "Result 2"(w2) -> ()
      n30 = local write "Result"(w2) -> ()
      n31 = call "Shutter_Init.vi"() -> ("error out"=w3:errorcluster, "ObjectPtr"=w4:i32)  [unwired: 2 in]
    }
    frame #1 {
      n32 = while {
        tunnel: w101 -> [w109]
        tunnel: w100 -> [w108]
        tunnel: w99 -> [w107]
        tunnel: w98 -> [w106]
        tunnel: w97 -> [w104]
        tunnel: w96 -> [w103]
        tunnel: w95 -> [w102]
        stop <- "stop" stop-if-true
        n33 = stacked-sequence {
          tunnel: w109 -> [w113 _ _ w203 _ _]
          tunnel: w108 -> [w112 _ _ w202 _ _]
          tunnel: w107 -> [w110 _ _ w201 _ _]
          tunnel: w106 -> [w111 _ _ w200 _ _]
          tunnel: w104 -> [_ _ _ w197 w326 _]
          tunnel: w103 -> [_ _ _ _ w325 _]
          tunnel: w102 -> [_ _ _ _ w324 _]
          frame #0 {
            n34 = case shown="True" "winspec" {
              tunnel: w113 -> [_ w118]
              tunnel: w112 -> [_ w117]
              tunnel: w111 -> [_ w116]
              tunnel: w110 -> [_ w115]
              frame False {
              }
              frame True {
                n35 = while {
                  tunnel: w118 -> [w123]
                  tunnel: w117 -> [w124]
                  tunnel: w116 -> [w132]
                  tunnel: w115 -> [w125]
                  stop <- w139 continue-if-true
                  n36 = stacked-sequence {
                    frame #0 {
                      # "This loop continuously updates the graph on the front with the image from the PIXIS"
                      n37 = local read "Camera Handle"() -> (w154:u32)
                      n38 = local read "# Images"() -> (w150:u16)
                      n39 = local read "error out"() -> (w153:errorcluster)
                      n40 = local read "Change to Raman Shift"() -> (w144:bool)
                      n41 = call "DataGrabber.vi"("# Images In"=w150, "Camera Handle"=w154, "error in (no error)"=w153) -> ("# Images Out"=w145:u16, "Camera Handle"=w152:u32, "Data"=w149:dbl[][], "error out"=w151:errorcluster)
                      n42 = case shown="True" w144 {
                        tunnel: [w156 w158] -> w142
                        tunnel: ["Pixel" ("X Scale.Name Label.Text") "Raman Shift (cm-1)" ("X Scale.Name Label.Text")] -> w140
                        frame False {
                          n43 = local read "Result"() -> (w156:dbl[])
                        }
                        frame True {
                          n44 = local read "Result 2"() -> (w158:dbl[])
                        }
                      }
                      n45 = Initialize Array(0.0, u32 1340) -> (w146:dbl[])
                      n46 = call "DataProcessor.vi"("PumpOffBkgd"=w146, "PumpOnBkgd"=w146, "Data"=w149, "# of Images"=w145) -> ("PumpOff"=w143:dbl[])  [unwired: 2 out]
                      n47 = local write "# Images"(w145) -> ()
                      n48 = Build Cluster Array(w142, w143) -> (w141:cluster{dbl, dbl}[])
                      n49 = property on="Spectra" class="XYGraph (strict)"("XScale.NameLbl.Text"=w140) -> ()  [unwired: 2 in, 2 out]
                      n50 = local write "Spectra"(w141) -> ()
                      n51 = local write "Camera Handle"(w152) -> ()
                      n52 = local write "error out"(w151) -> ()
                    }
                    frame #1 {
                      n53 = stacked-sequence {
                        frame #0 {
                          # "Select Cursor 0"
                          n54 = property on="Spectra" class="XYGraph (strict)"("Active Cursor"=0) -> ()  [unwired: 2 in, 2 out]
                        }
                        frame #1 {
                          # "Record the Y position of cursor 0"
                        }
                        frame #2 {
                          # "Select Cursor 1"
                          n55 = property on="Spectra" class="XYGraph (strict)"("Active Cursor"=1) -> ()  [unwired: 2 in, 2 out]
                        }
                        frame #3 {
                          # "Calculate the Gain"
                          n56 = property on="Spectra" class="XYGraph (strict)"() -> ("Cursor.Cursor Position:Cursor Y"=w166:dbl)  [unwired: 2 in, 2 out]
                          n57 = local read "cursor y 2"() -> (w165:dbl)
                          n58 = Subtract(x=w166, y=w165) -> (x-y=w162:dbl)
                          n59 = Absolute Value(x=w162) -> (abs(x)=w164:dbl)
                          n60 = Multiply(x=w164, y=1) -> (x*y=w161:dbl)
                          n61 = local write "Gain"(w161) -> ()
                        }
                      }
                    }
                  }
                  n62 = local read "winspec"() -> (w139:bool)
                  n63 = Boolean To (0,1)(Boolean="PUMP") -> (0, 1=w137:i16)
                  n64 = Multiply(x="Step Size (micro meter)", y=10.0) -> (x*y=w120:dbl)
                  n65 = Add(x=w137, y=i16 1) -> (x+y=w126:i16)
                  n66 = Round To Nearest(number=w120) -> (nearest integer value=w119:dbl)
                  n67 = And(x="MOVE", y=w139) -> (x .and. y?=w133:bool)
                  n68 = call "Pico_move_new.vi"("Motor"=w126, "CmdLib Out"=w123, "DeviceKey Out"=w124, "Start Position"="Start Position", "Boolean 2"="GO", "Relative Steps"=w119, "Boolean"=w133, "error out"=w132, "Device Address Out"=w125) -> ("CmdLib Out"=→"CmdLib Out":refnum<k24>, "DeviceKey Out"=→"DeviceKey Out":string, "Device Address Out"=→"Device Address Out":i32, "error out 2"=→"error out 2":errorcluster)  [unwired: 3 in]
                }
              }
            }
          }
          frame #1 {
            n69 = case shown="True" "Bkgnd" {
              frame False {
              }
              frame True {
                # "Process the Data"
                # "Get the data!"
                # "Display the Raman Pump on graph on the Front Panel and store data"
                n70 = local read "Camera Handle"() -> (w181:u32)
                n71 = local read "# Images"() -> (w176:u16)
                n72 = local read "error out"() -> (w180:errorcluster)
                n73 = local read "Change to Raman Shift"() -> (w169:bool)
                n74 = call "DataGrabber.vi"("# Images In"=w176, "Camera Handle"=w181, "error in (no error)"=w180) -> ("# Images Out"=w173:u16, "Camera Handle"=w179:u32, "Data"=w177:dbl[][], "error out"=w178:errorcluster)
                n75 = local write "Camera Handle"(w179) -> ()
                n76 = local write "error out"(w178) -> ()
                n77 = local write "# Images"(w173) -> ()
                n78 = case shown="True" w169 {
                  tunnel: [w185 w187] -> w172
                  tunnel: ["Pixel" ("X Scale.Name Label.Text") "Raman Shift (cm-1)" ("X Scale.Name Label.Text")] -> w168
                  frame False {
                    n79 = local read "Result"() -> (w185:dbl[])
                  }
                  frame True {
                    n80 = local read "Result 2"() -> (w187:dbl[])
                  }
                }
                n81 = Initialize Array(0.0) -> (w174:dbl[])  [unwired: 1 in]
                n82 = call "DataProcessor.vi"("PumpOffBkgd"=w174, "PumpOnBkgd"=w174, "Data"=w177, "# of Images"=w173) -> ("PumpOff"=→"Bkgndoff":dbl[], "PumpOn"=→"Bkgndon":dbl[], "Raman"=w171:dbl[])
                n83 = Build Cluster Array(w172, w171) -> (w170:cluster{dbl, dbl}[])
                n84 = property on="Spectra" class="XYGraph (strict)"("XScale.NameLbl.Text"=w168) -> ()  [unwired: 2 in, 2 out]
                n85 = local write "Spectra"(w170) -> ()
              }
            }
          }
          frame #2 {
            n86 = case shown="True" "Callibration" {
              frame False {
              }
              frame True {
                n87 = for {
                  N: 1340 -> [_]
                  tunnel: [w196] -> w195 mode=indexing
                  i -> [w196]
                }
                n88 = call "cal.vi"("array"=w195, "Laser Wavelength"="Laser Wavelength (nm)", "Wave Number"="Shift", "Pixel"="Pixel") -> ("array 2"=→"Result":dbl[], "Result"=→"Result 2":dbl[])  [unwired: 6 in]
              }
            }
          }
          frame #3 {
            n89 = Compound Arithmetic op=OR("Acquire", "Focus") -> (w204:bool)
            n90 = case shown="True" w204 {
              selector: w204 -> [_ w210]
              tunnel: w203 -> [_ w209]
              tunnel: w202 -> [_ w208]
              tunnel: w201 -> [_ w207]
              tunnel: w200 -> [_ w206]
              tunnel: w197 -> [_ w205]
              frame False {
              }
              frame True {
                n91 = while {
                  tunnel: w210 -> [w244]
                  tunnel: w209 -> [w236]
                  tunnel: w208 -> [w235]
                  tunnel: w207 -> [w234]
                  tunnel: w206 -> [w233]
                  tunnel: w205 -> [w212]
                  stop <- w211 continue-if-true
                  n92 = stacked-sequence {
                    seq-local: [w255 _ _ _] -> [_ w279 _ _]
                    seq-local: [w261 _ _ _] -> [_ w276 _ _]
                    frame #0 {
                      n93 = local read "Camera Handle"() -> (w265:u32)
                      n94 = local read "# Images"() -> (w266:u16)
                      n95 = local read "error out"() -> (w264:errorcluster)
                      n96 = local read "Change to Raman Shift"() -> (w251:bool)
                      n97 = call "DataGrabber.vi"("# Images In"=w266, "Camera Handle"=w265, "error in (no error)"=w264) -> ("# Images Out"=w255:u16, "Camera Handle"=w262:u32, "Data"=w261:dbl[][], "error out"=w263:errorcluster)
                      n98 = case shown="False" w251 {
                        tunnel: [w268 w270] -> w249
                        tunnel: ["Pixel" ("X Scale.Name Label.Text") "Raman Shift (cm-1)" ("X Scale.Name Label.Text")] -> w252
                        frame False {
                          n99 = local read "Result"() -> (w268:dbl[])
                        }
                        frame True {
                          n100 = local read "Result 2"() -> (w270:dbl[])
                        }
                      }
                      n101 = local write "Camera Handle"(w262) -> ()
                      n102 = local write "error out"(w263) -> ()
                      n103 = Initialize Array(0.0, u32 1340) -> (w258:dbl[])
                      n104 = local write "# Images"(w255) -> ()
                      n105 = call "DataProcessor.vi"("PumpOffBkgd"=w258, "PumpOnBkgd"=w258, "Data"=w261, "# of Images"=w255) -> ("PumpOff"=w256:dbl[], "PumpOn"=w257:dbl[], "Raman"=w253:dbl[])
                      n106 = local write "Off"(w256) -> ()
                      n107 = property on="Spectra" class="XYGraph (strict)"("XScale.NameLbl.Text"=w252) -> ()  [unwired: 2 in, 2 out]
                      n108 = local write "On"(w257) -> ()
                      n109 = case shown="True" "Flip Spectra" {
                        tunnel: [w271 w272] -> w250
                        tunnel: w253 -> [w271 w273]
                        frame False {
                        }
                        frame True {
                          # "Flip Displayed Spectra"
                          n110 = Reciprocal(x=w273) -> (1/x=w272:dbl[])
                        }
                      }
                      n111 = local write "Raman"(w253) -> ()
                      n112 = Build Cluster Array(w249, w250) -> (w248:cluster{dbl, dbl}[])
                      n113 = local write "Spectra"(w248) -> ()
                    }
                    frame #1 {
                      w283 = 2
                      n114 = Initialize Array(0.0, u32 1340) -> (w287:dbl[])
                      n115 = Initialize Array(0.0, u32 1340) -> (w288:dbl[])
                      n116 = Subtract(x=w279, y=u16 10) -> (x-y=w278:u16)
                      n117 = Divide(x=w279, y=w283) -> (x/y=w284:dbl)
                      n118 = Delete From Array(array=w276, length=10, index (row)=0) -> (array with subset deleted=w275:dbl[][])  [unwired: 1 in, 1 out]
                      n119 = for {
                        N: w278 -> [_]
                        tunnel: w275 -> [w299]
                        shift-right: [w297] -> w286
                        shift-left: w288 -> [w298]
                        shift-right: [w295] -> w285
                        shift-left: w287 -> [w296]
                        tunnel: w283 -> [w294]
                        i -> [w293]
                        n120 = Quotient & Remainder(x=w293, y=w294) -> (x-y*floor(x/y)=w301:i32)  [unwired: 1 out]
                        n121 = Equal To 0?(x=w301) -> (x = 0?=w300:bool)
                        n122 = case shown="True" w300 {
                          tunnel: w299 -> [w306 w313]
                          tunnel: w298 -> [w307 w311]
                          tunnel: [w307 w310] -> w297
                          tunnel: w296 -> [w305 w309]
                          tunnel: [w303 w309] -> w295
                          tunnel: w293 -> [w302 w308]
                          frame False {
                            # "Raman Pump Off\nOdd Images"
                            n123 = Index Array(array=w306, index (row)=w302) -> (element=w304:dbl[])  [unwired: 1 in]
                            n124 = Add(x=w304, y=w305) -> (x+y=w303:dbl[])
                          }
                          frame True {
                            # "Raman pump on\nEven Images"
                            n125 = Index Array(array=w313, index (row)=w308) -> (element=w312:dbl[])  [unwired: 1 in]
                            n126 = Add(x=w312, y=w311) -> (x+y=w310:dbl[])
                          }
                        }
                      }
                      n127 = Divide(x=w286, y=w284) -> (x/y=w281:dbl[])
                      n128 = Divide(x=w285, y=w284) -> (x/y=w282:dbl[])
                      n129 = Divide(x=w281, y=w282) -> ()  [unwired: 1 out]
                    }
                    frame #2 {
                      # "Calculate the Gain based on the two cursors on the graph"
                      n130 = stacked-sequence {
                        frame #0 {
                          # "Select Cursor 0"
                          n131 = property on="Spectra" class="XYGraph (strict)"("Active Cursor"=0) -> ()  [unwired: 2 in, 2 out]
                        }
                        frame #1 {
                          # "Record the Y position of cursor 0"
                          n132 = property on="Spectra" class="XYGraph (strict)"() -> ("Cursor.Cursor Position:Cursor Y"=→"cursor y":dbl)  [unwired: 2 in, 2 out]
                        }
                        frame #2 {
                          # "Select Cursor 1"
                          n133 = property on="Spectra" class="XYGraph (strict)"("Active Cursor"=1) -> ()  [unwired: 2 in, 2 out]
                        }
                        frame #3 {
                          # "Calculate the Gain"
                          n134 = property on="Spectra" class="XYGraph (strict)"() -> ("Cursor.Cursor Position:Cursor Y"=w317:dbl)  [unwired: 2 in, 2 out]
                          n135 = local read "cursor y"() -> (w322:dbl)
                          n136 = Subtract(x=w317, y=w322) -> (x-y=w319:dbl)
                          n137 = Absolute Value(x=w319) -> (abs(x)=w321:dbl)
                          n138 = Multiply(x=w321, y=100) -> (x*y=→"Gain":dbl)
                        }
                      }
                    }
                    frame #3 {
                      n139 = Wait (ms)(milliseconds to wait=50) -> ()  [unwired: 1 out]
                    }
                  }
                  n140 = call <instrlib>:"_subvi_LivePos_Main.vi"("xCommand"="xCommand", "yCommand"="yCommand", "zCommand"="zCommand", "handle"=w212, "commandZ"="commandZ", "commandY"="commandY", "commandX"="commandX") -> ("xRead"=w223:dbl, "yRead"=w222:dbl, "zRead"=w221:dbl, "counter"=w213:u32)  [unwired: 1 in, 8 out]
                  n141 = Equal To 0?(x=w213) -> (x = 0?=w214:bool)
                  n142 = case shown="True" w214 {
                    tunnel: w223 -> [_ w247]
                    tunnel: w222 -> [_ w246]
                    tunnel: w221 -> [_ w245]
                    frame False {
                    }
                    frame True {
                      "xRead" <- w247
                      "yRead" <- w246
                      "zRead" <- w245
                    }
                  }
                  n143 = local read "Focus"() -> (w211:bool)
                  n144 = local read "Step Size (micro meter)"() -> (w227:dbl)
                  n145 = local read "Start Position"() -> (w238:i32)
                  n146 = local read "MOVE"() -> (w240:bool)
                  n147 = local read "PUMP"() -> (w241:bool)
                  n148 = local read "GO"() -> (w232:bool)
                  n149 = Boolean To (0,1)(Boolean=w241) -> (0, 1=w243:i16)
                  n150 = Add(x=w243, y=i16 1) -> (x+y=w239:i16)
                  n151 = And(x=w240, y=w244) -> (x .and. y?=w237:bool)
                  n152 = Multiply(x=w227, y=10.0) -> (x*y=w225:dbl)
                  n153 = Round To Nearest(number=w225) -> (nearest integer value=w224:dbl)
